vi "Close API Reference.vi"(8 "error in (no error)":errorcluster, 11 "Execution API In":refnum<class "Execution API.lvclass">) -> (0 "error out":errorcluster)   [LabVIEW 2020, in "Execution API.lvclass"]
doc: "Closes the API reference. Please note that any Event Registrations obtained from the Register for Events.vi will need to be unregistered for."
uses:
  Execution API.lvclass
  Execution API.lvclass/Execution API.ctl
  Framework/Plugin/Plugin.lvclass
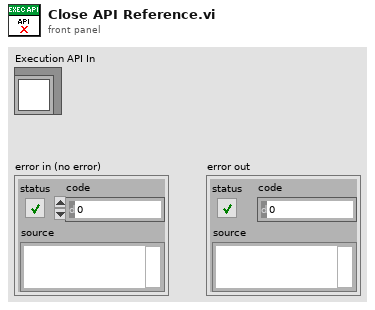
[diagram p1: front panel]
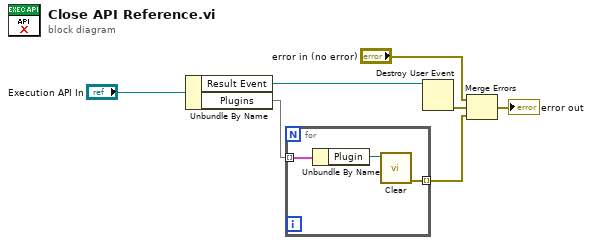
[diagram p0: block diagram]
diagram:
  n1 = Unbundle By Name("Execution API In") -> ("Result Event"=w3:refnum<user-event>, "Plugins"=w4:map{string, refnum<class "Plugin.lvclass">})
  n2 = for {
    tunnel: w4 -> [w10] mode=indexing
    tunnel: [w8] -> w1 mode=indexing
    n3 = Unbundle By Name(w10) -> ("Plugin"=w9:refnum<class "Plugin.lvclass">)
    n4 = call-dynamic "Clear.vi"("Plugin in"=w9) -> ("error out"=w8:errorcluster)  [unwired: 10 in]
  }
  n5 = Destroy User Event(user event=w3) -> (error out=w2:errorcluster)  [unwired: 1 in]
  n6 = Merge Errors("error in (no error)", w2, w1) -> (→"error out":errorcluster)
